vi "Set configuration chain.vi"(8 "error in (no error)":errorcluster, 9 "class names":string[](array[string]), 10 "configuration":variant[](array[variant]), 11 "Cascade in":refnum<class "Cascade.lvclass">) -> (0 "error out":errorcluster, 3 "Cascade out":refnum<class "Cascade.lvclass">)   [LabVIEW 2012, in "Cascade.lvclass"]
uses:
  Cascade.lvclass
  <vilib>/Distrio/Murmex/Murmex/Murmex.lvclass
  Cascade.lvclass/Cascade.ctl
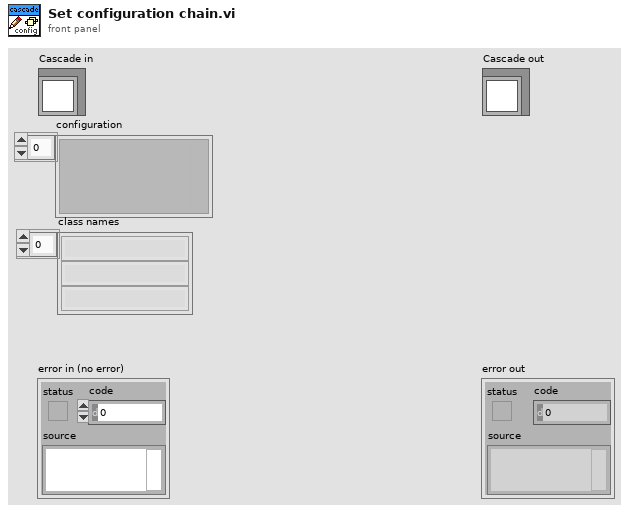
[diagram p1: front panel]
types:
  T1 = typedef "Cascade.lvclass/configuration.ctl" = cluster{"Trigger mode":T2, "Trigger Edge":T3, "Temperature":dbl, "Number of cleans":u16, "LUT":path, "stage component":string, "Background image":path, "Circular buffer frames":u32, "Electro-multiplying?":bool, "Buffer mode":T4, "micron equivalent of pixel":dbl[unit], "max x pixel displacement":dbl, "min x pixel displacement":dbl, "max pixel discrepancy":dbl, "max y pixel displacement":dbl, "min y pixel displacement":dbl, "brightness threshold":sgl, "Binarization parameters":T5, "Gaussian blur parameters":T6, "Edge and object Parameters":T7, "Registration method":T8, "saturation limit":dbl, "max physical displacement":dbl[unit], "min physical displacement":dbl[unit], "image conversion shifts":i32}
  T2 = typedef "Trigger mode.ctl" = i16
  T3 = typedef "Cascade.lvclass/Trigger edge.ctl" = u32
  T4 = typedef "Buffer mode.ctl" = i16
  T5 = typedef "BinarizationParameters.ctl" = cluster{"threshold percentage":dbl, "equalize?":bool, "Method (clustering)":i32}
  T6 = typedef "Gaussian blur parameters.ctl" = cluster{"large sigma":sgl, "small sigma":sgl, "equalize?":bool}
  T7 = typedef "Edge and object parameters.ctl" = cluster{"Canny Edge Parameters":cluster{"Sigma":sgl, "HThresh":sgl, "LThres":sgl, "WindowSize":i32}, "Smoothing parameters":cluster{"X Size":i32, "Y Size":i32, "% Tolerance":i32}, "Dilation iteration":i32, "Object recognition parameters":cluster{"Objects":u16, "Threshold":i32, "Reject Border":bool, "Fill Holes":bool, "Min Object Size":bool, "Min Size":i32, "Max Object Size":bool, "Max Size":i32, "Show Search Area":bool, "Show Center":bool, "Show Bounding Box":bool}}
  T8 = typedef "Registration method.ctl" = enum16{"Binarization", "Difference of Gaussians", "Edges Detection", "Gaussians and Binarization", "Edges and Gaussians", "Edges and Binarization", "All"}
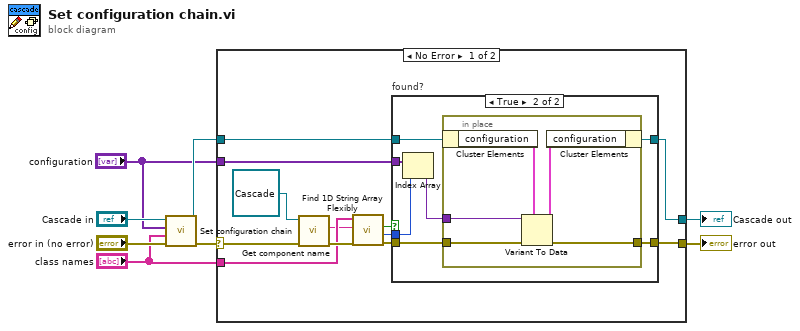
[diagram p0: block diagram]
diagram:
  n1 = call-parent "Set configuration chain.vi"("error in (no error)"="error in (no error)", "class names"="class names", "configuration"="configuration", "Murmex in"="Cascade in") -> ("error out"=w6:errorcluster, "Murmex out"=w5:refnum<class "Cascade.lvclass">)  [unwired: 6 in]
  n2 = case shown="No Error" w6 {
    selector: w6 -> [w20 w36]
    tunnel: w5 -> [w14 w35]
    tunnel: [w9 w36] -> w4
    tunnel: [w10 w35] -> w3
    tunnel: "class names" -> [w17 _]
    tunnel: "configuration" -> [w13 _]
    frame No Error {
      n3 = call <vilib>:"Get component name.vi"("error in (no error)"=w20, "Murmex in"=refnum<class "Cascade.lvclass"> refnum ("Cascade.lvclass")) -> ("error out"=w18:errorcluster, "component name"=w16:string)  [unwired: 7 in, 1 out]
      n4 = call <vilib>:"Find 1D String Array Flexibly.vi"("error in (no error)"=w18, "element"=w16, "array"=w17) -> ("error out"=w15:errorcluster, "index of element"=w11:i32, "found?"=w12:bool)  [unwired: 6 in]
      n5 = case "found?" shown="True" w12 {
        tunnel: w13 -> [_ w29]
        tunnel: w14 -> [w22 w27]
        tunnel: [w22 w26] -> w10
        tunnel: [w21 w25] -> w9
        tunnel: w15 -> [w21 w24]
        tunnel: w11 -> [_ w23]
        frame False {
        }
        frame True {
          n6 = Index Array(array=w29, index=w23) -> (element=w28:variant)
          n7 = in-place {
            in-place-border: w28 -> [w34]
            in-place-border: w24 -> [w32]
            in-place-border: [w30] -> w25
            n8 = in-place-cluster #1(w27) -> ("configuration"=w33:T1)
            n9 = Variant To Data(error in=w32, type=w33, Variant=w34) -> (data=w31:T1, error out=w30:errorcluster)
            n10 = in-place-cluster #1("configuration"=w31) -> (w26:refnum<class "Cascade.lvclass">)
          }
        }
      }
    }
    frame Error {
    }
  }
  "error out" <- w4
  "Cascade out" <- w3
